vi "błąd długości.vi"(4 "błąd długości":errorcluster) -> (1 "Błędy długości":string)   [LabVIEW 2015, in "Biblioteka moduł map v3.lvlib" / "Konwersja wsp.lvlib" / "Obsługa błędów.lvlib"]
doc: "SubVI ma za zadanie sprawdzić czy wystąpiły błędy związane z długością. Jeżli tak to ma dopisać tekst informujący o błędach związanych z długością geograficzną."
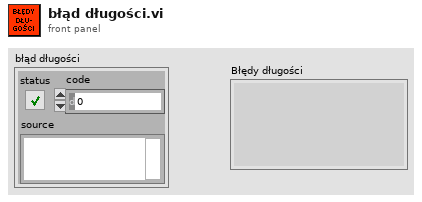
[diagram p1: front panel]
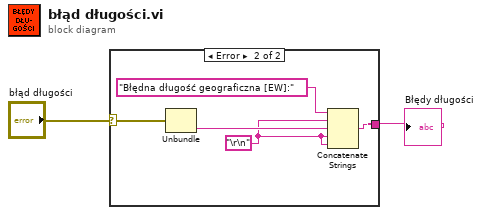
[diagram p0: block diagram]
diagram:
  n1 = case shown="Error" "błąd długości" {
    selector: "błąd długości" -> [_ w6]
    tunnel: [_ w4] -> w1
    frame No Error {
    }
    frame Error {
      w3 = "\r\n"
      n2 = Unbundle(w6) -> ("source"=w5:string)  [unwired: 2 out]
      n3 = Concatenate Strings("Błędna długość geograficzna [EW]:" ("source"), w3, w5, w3, w3) -> (w4:string)
    }
  }
  "Błędy długości" <- w1
